vi "DSF.Engine.Pointer.DBL.Get Channel Count.vi"(11 "DBL Buffer in":refnum<class "DSF.Engine.Pointer.DBL.lvclass">) -> (2 "channel count":u64, 3 "DBL Buffer out":refnum<class "DSF.Engine.Pointer.DBL.lvclass">)   [LabVIEW 2017, in "DSF.Engine.lvlib" / "DSF.Engine.Pointer.DBL.lvclass"]
uses:
  DSF.Engine.Pointer.DBL.lvclass
  DSF.Engine.Pointer.DBL.lvclass/DSF.Engine.Pointer.DBL.ctl
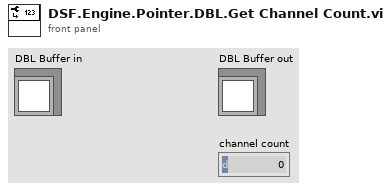
[diagram p1: front panel]
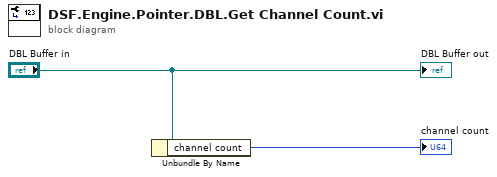
[diagram p0: block diagram]
diagram:
  n1 = Unbundle By Name("DBL Buffer in") -> ("channel count"=→"channel count":u64)
  "DBL Buffer out" <- "DBL Buffer in"
